vi "Write Camera Status.vi"(8 "error in (no error)":errorcluster, 10 "Camera Status":T1, 11 "CCDCamera in":refnum<class "CCDCamera.lvclass">) -> (0 "error out":errorcluster, 3 "CCDCamera out":refnum<class "CCDCamera.lvclass">)   [LabVIEW 2018, in "CCDCamera.lvclass"]
uses:
  CCDCamera.lvclass
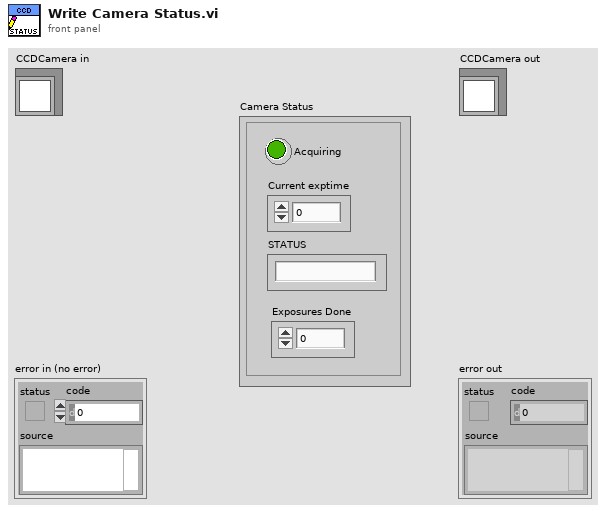
[diagram p1: front panel]
types:
  T1 = cluster{"Acquiring":bool, "Current exptime":sgl, "STATUS":string, "Exposures Done":u16}
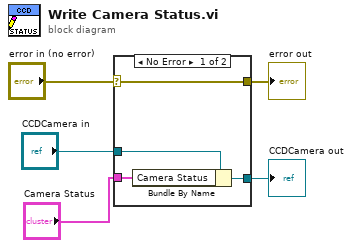
[diagram p0: block diagram]
diagram:
  n1 = case shown="No Error" "error in (no error)" {
    selector: "error in (no error)" -> [w9 w10]
    tunnel: [w9 w10] -> w4
    tunnel: [w7 w11] -> w2
    tunnel: "CCDCamera in" -> [w8 w11]
    tunnel: "Camera Status" -> [w6 _]
    frame No Error {
      n2 = Bundle By Name(cluster=w8, "Camera Status"=w6) -> (w7:refnum<class "CCDCamera.lvclass">)
    }
    frame Error {
    }
  }
  "error out" <- w4
  "CCDCamera out" <- w2
